vi "Stop (Jeevan Anga's conflicted copy 2013-04-07).vi"   [LabVIEW 2011]
uses:
  jeevan/Global Variables.vi
types:
  T1 = cluster{"Drive Value Output String":string, "Steer Value Output String":string, "Error Out":errorcluster}
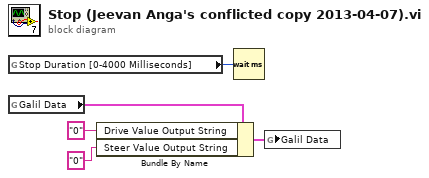
[diagram p0: block diagram]
diagram:
  n1 = global read "Global Variables.vi" "Stop Duration [0-4000 Milliseconds]"() -> (w1:u32)
  n2 = global read "Global Variables.vi" "Galil Data"() -> (w3:T1)
  n3 = Bundle By Name(cluster=w3, "Drive Value Output String"="0", "Steer Value Output String"="0") -> (w2:T1)
  n4 = Wait (ms)(milliseconds to wait=w1) -> ()  [unwired: 1 out]
  n5 = global write "Global Variables.vi" "Galil Data"(w2) -> ()
